vi "Launch Action - TDMS Defragment.vi"(8 "error in (no error)":errorcluster, 11 "file path":path) -> (0 "error out":errorcluster)   [LabVIEW 2021, in "XNET-CAN-Signal-Logger.lvlib"]
uses:
  XNET-CAN-Signal-Logger.lvlib
  Action - TDMS Defragment.vi
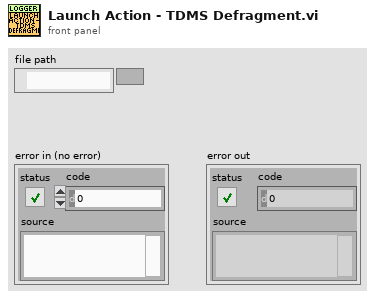
[diagram p1: front panel]
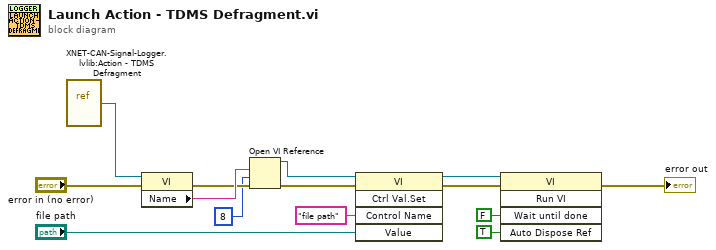
[diagram p0: block diagram]
diagram:
  n1 = vi-ref "XNET-CAN-Signal-Logger.lvlib:Action - TDMS Defragment.vi"() -> (w14:refnum<vi>)
  n2 = property class="VI"(reference=w14, error in="error in (no error)") -> (error out=w12:errorcluster, "Name"=w13:string)  [unwired: 1 out]
  n3 = Open VI Reference(vi path=w13, options=8, error in (no error)=w12) -> (vi reference=w11:refnum<vi>, error out=w10:errorcluster)  [unwired: 3 in]
  n4 = invoke class="VI" method="Ctrl Val.Set"(reference=w11, error in=w10, "Control Name"="file path", "Value"="file path") -> (reference out=w6:refnum<vi>, error out=w5:errorcluster)  [unwired: 1 in, 3 out]
  n5 = invoke class="VI" method="Run VI"(reference=w6, error in=w5, "Wait until done"=FALSE ("Wait Until Done"), "Auto Dispose Ref"=TRUE ("Auto Dispose Reference")) -> (error out=→"error out":errorcluster)  [unwired: 1 in, 4 out]
